vi "Set IO Level.vi"(8 "error in (no error)":errorcluster, 10 "iLevel":i32, 11 "index":i32) -> (0 "error out":errorcluster, 3 "function return":u32)   [LabVIEW 2014, in "atmcd32d.lvlib"]
doc: "unsigned int WINAPI SetIOLevel(int index, int iLevel);"
uses:
  atmcd32d.lvlib
  atmcd32d.dll
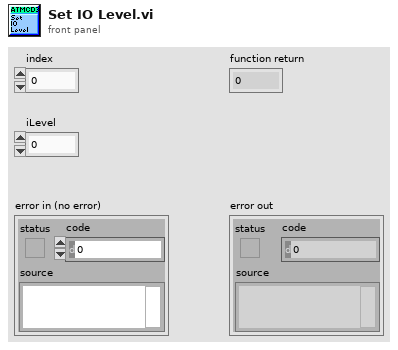
[diagram p1: front panel]
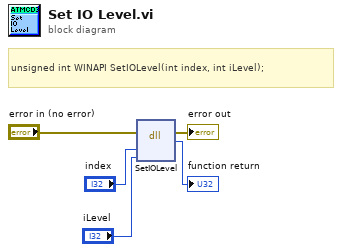
[diagram p0: block diagram]
diagram:
  # "unsigned int WINAPI SetIOLevel(int index, int iLevel);"
  n1 = dll-call lib="C:/Users/Bakir/Documents/Lambda2-Testing/lib/Andorlib/atmcd32d.*" fn="SetIOLevel"(error in="error in (no error)", "index"="index", "iLevel"="iLevel") -> (error out=→"error out":errorcluster, →"function return":u32)  [unwired: 4 in, 1 out]
